vi "InvokeMatlabEvent.vi"(0 "ExpID":string, 5 "Event":T1 items=["[FromStringName]", "updateExpParameter", "invokeMethod"], 7 "Data":variant, 9 "event by name":string, 11 "error in (no error)":errorcluster, 12 "Invoke?":bool=TRUE) -> (15 "error out":errorcluster)   [LabVIEW 2017]
uses:
  Types/MatlabEventNameTypes.ctl
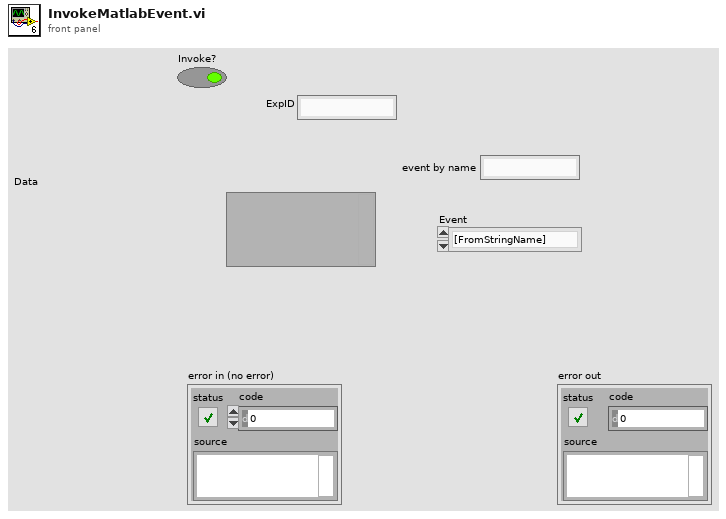
[diagram p1: front panel]
types:
  T1 = typedef "MatlabEventNameTypes.ctl" = u16
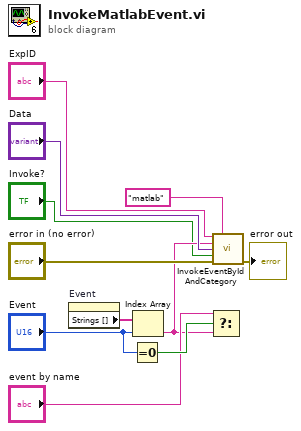
[diagram p0: block diagram]
diagram:
  n1 = property on="Event" class="Ring (strict)"() -> ("Strings []"=w6:string[])  [unwired: 2 in, 2 out]
  n2 = Equal To 0?(x="Event") -> (x = 0?=w4:bool)
  n3 = Index Array(array=w6, index="Event") -> (element=w2:string)
  n4 = Select(t="event by name", s=w4, f=w2) -> ()  [unwired: 1 out]
  n5 = call "InvokeEventByIdAndCategory.vi"("ID"="ExpID", "Category"="matlab", "eventName"=w2, "Data"="Data", "Invoke? (t)"="Invoke?", "error in (no error)"="error in (no error)") -> ("error out"=→"error out":errorcluster)  [unwired: 9 in]
